vi "TDMS2TDMCheckName.vi"(2 "Name Type":T1, 7 "Name":string) -> (8 "Name Out":string)   [LabVIEW 2017]
doc: "This VI checks for illegal characters in channel group, channel, or property names. If illegal characters are found, the name is coerced to one that fits the proper TDM storage format."
uses:
  <vilib>/Utility/tdmsutil.llb/TDMS2TDMNameType.ctl
  <vilib>/Utility/tdmsutil.llb/TDMS2TDMLogIllegalName.vi
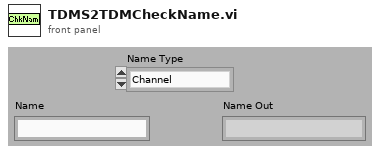
[diagram p1: front panel]
types:
  T1 = typedef "TDMS2TDMNameType.ctl" = enum16{"Channel", "Property"}
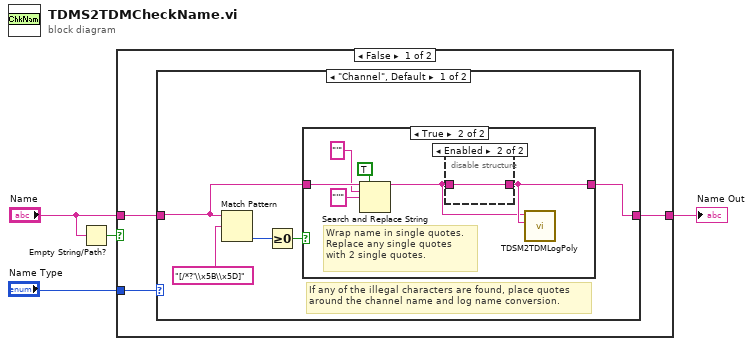
[diagram p0: block diagram]
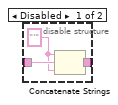
[diagram p3: hidden frame]
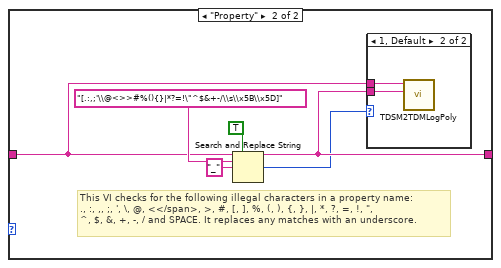
[diagram p4: hidden frame]
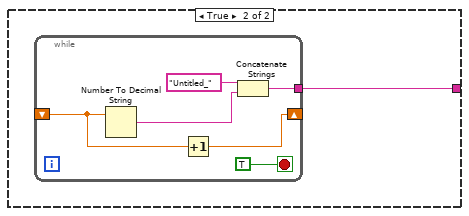
[diagram p6: hidden frame]
diagram:
  n1 = Empty String/Path?(string/path="Name") -> (empty?=w1:bool)
  n2 = case shown="False" w1 {
    tunnel: [w7 w32] -> w4
    tunnel: "Name" -> [w6 _]
    tunnel: "Name Type" -> [w5 _]
    frame False {
      n3 = case shown="\"Channel\", Default" w5 {
        tunnel: [w12 w29] -> w7
        tunnel: w6 -> [w8 w25]
        frame "Channel", Default {
          # "If any of the illegal characters are found, place quotes\naround the channel name and log name conversion."
          n4 = Match Pattern(string=w8, regular expression="[/*?'\\x5B\\x5D]" ("search string")) -> (offset past match=w10:i32)  [unwired: 1 in, 3 out]
          n5 = Greater Or Equal To 0?(x=w10) -> (x >= 0?=w9:bool)
          n6 = case shown="True" w9 {
            tunnel: w8 -> [w13 w18]
            tunnel: [w13 w19] -> w12
            frame False {
            }
            frame True {
              # "Wrap name in single quotes.\nReplace any single quotes\nwith 2 single quotes."
              n7 = Search and Replace String(replace all?=TRUE ("replace all? (F)"), input string=w18, search string="'" ("string"), replace string="''" ("replace string (\"\")")) -> (result string=w16:string)  [unwired: 4 in, 3 out]
              n8 = disable-structure shown="Enabled" {
                disable-tunnel: [w22 w23] -> w19
                disable-tunnel: w16 -> [w21 w23]
                frame Disabled {
                  w20 = "'" ("replace string (\"\")")
                  n9 = Concatenate Strings(w20, w21, w20) -> (w22:string)
                }
                frame Enabled {
                }
              }
              n10 = call-poly <vilib>:"TDSM2TDMLogPoly.vi"("New Name"=w19, "Original Name"=w16) -> ()  [unwired: 9 in, 1 out]
            }
          }
        }
        frame "Property" {
          # "This VI checks for the following illegal characters in a property name:\n., :, ,, ;, ', \\, @, <</span>, >, #, [, ], %, (, ), {, }, |, *, ?, =, !, \",\n^, $, &, +, -, / and SPACE. It replaces any matches with an underscore."
          n11 = Search and Replace String(replace all?=TRUE ("replace all? (F)"), input string=w25, search string="[.:,;'\\@<>>#%(){}|*?=!\"^$&+-/\\s\\x5B\\x5D]", replace string="_" ("replace string (\"\")")) -> (result string=w29:string, number of replacements=w24:i32)  [unwired: 4 in, 2 out]
          n12 = case shown="1, Default" w24 {
            tunnel: w29 -> [_ w31]
            tunnel: w25 -> [_ w30]
            frame 0 {
            }
            frame 1, Default {
              n13 = call-poly <vilib>:"TDSM2TDMLogPoly.vi"("New Name"=w31, "Original Name"=w30) -> ()  [unwired: 9 in, 1 out]
            }
          }
        }
      }
    }
    frame True {
      n14 = while {
        shift-right: [w35] -> _
        shift-left: _ -> [w36]
        tunnel: [w34] -> w32
        stop <- TRUE stop-if-true
        n15 = Number To Decimal String(number=w36) -> (decimal integer string=w37:string)  [unwired: 1 in]
        n16 = Increment(x=w36) -> (x+1=w35:dbl)
        n17 = Concatenate Strings("Untitled_" ("string"), w37) -> (w34:string)
      }
    }
  }
  "Name Out" <- w4
